vi "Build Data Frame.vi"(0 "RFFE RegWrite Command in":refnum<class "RFFE RegWrite Command.lvclass">, 11 "error in (no error)":errorcluster) -> (4 "RFFE RegWrite Command out":refnum<class "RFFE RegWrite Command.lvclass">, 6 "Data Frame":u8[](array[numeric]), 15 "error out":errorcluster)   [LabVIEW 2018, in "MIPI RFFE API.lvlib" / "RFFE RegWrite Command.lvclass"]
uses:
  RFFE RegWrite Command.lvclass
  C:/Users/semoore/Projects/mipi-rffe-labview-oop/Standard Command/RFFE Standard Command.lvclass
  Standard Command/RFFE Standard Command.lvclass/RFFE Standard Command.ctl
  Standard Command/Get Register Data.vi
  MIPI RFFE API.lvlib
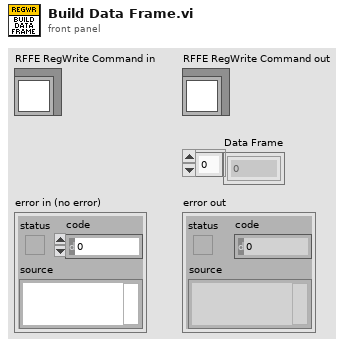
[diagram p1: front panel]
types:
  T1 = typedef "RFFE Commands.lvlib/Register Data.ctl" = u8
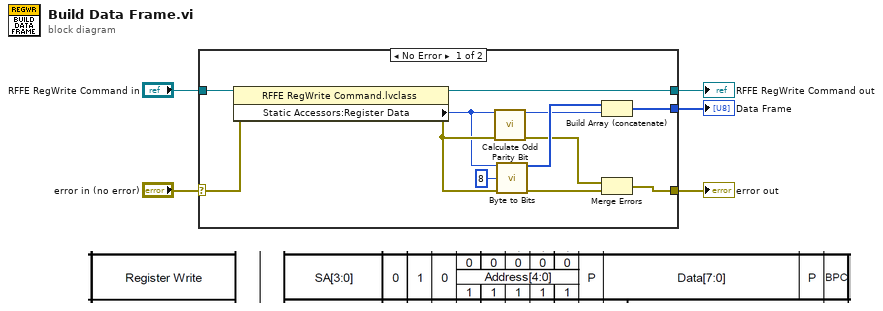
[diagram p0: block diagram]
diagram:
  n1 = case shown="No Error" "error in (no error)" {
    selector: "error in (no error)" -> [w8 w19]
    tunnel: [w15 w19] -> w3
    tunnel: "RFFE RegWrite Command in" -> [w11 w18]
    tunnel: [w10 _] -> w4
    tunnel: [w9 w18] -> w1
    frame No Error {
      n2 = property class="RFFE RegWrite Command.lvclass"(reference=w11, error in=w8) -> (reference out=w9:refnum<class "RFFE RegWrite Command.lvclass">, error out=w7:errorcluster, "Static Accessors:Register Data"=w6:T1)
      n3 = call "Calculate Odd Parity Bit.vi"("Byte"=w6, "error in (no error)"=w7) -> ("Odd Parity Bit"=w14:u8, "error out"=w13:errorcluster)  [unwired: 12 in]
      n4 = call "Byte to Bits.vi"("Byte"=w6, "Bit Width"=8, "error in (no error)"=w7) -> ("Bits"=w16:u8[], "error out"=w12:errorcluster)  [unwired: 11 in]
      n5 = Build Array (concatenate)(w16, w14) -> (w10:u8[])
      n6 = Merge Errors(w13, w12) -> (w15:errorcluster)
    }
    frame Error {
    }
  }
  "error out" <- w3
  "RFFE RegWrite Command out" <- w1
  "Data Frame" <- w4
